vi "例7-6（1）.vi"() -> ()   [LabVIEW 2019]
uses:
  <vilib>/Analysis/NI_AALBase.lvlib
panel:
  in  "停止":bool
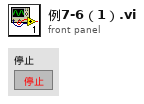
[diagram p1: front panel]
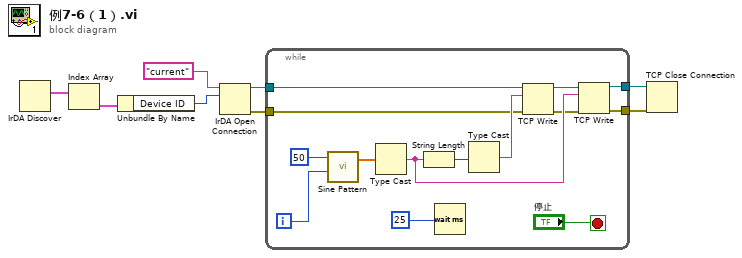
[diagram p0: block diagram]
diagram:
  n1 = IrDA Discover() -> (2:w8:cluster{"Device ID":u32, "Device Name":string}[])  [unwired: 1 in, 2 out]
  n2 = Index Array(array=w8) -> (element=w7:cluster{"Device ID":u32, "Device Name":string})  [unwired: 1 in]
  n3 = Unbundle By Name(w7) -> ("Device ID"=w6:u32)
  n4 = IrDA Open Connection(10:w6, 11:"current" ("服务名称")) -> (0:w2:errorcluster, 3:w4:refnum<k19>)  [unwired: 2 in]
  n5 = while {
    tunnel: w4 -> [w15]
    tunnel: [w13] -> w3
    tunnel: w2 -> [w12]
    tunnel: [w10] -> w1
    i -> [w20]
    stop <- "停止" stop-if-true
    n6 = call <vilib>:"Sine Pattern.vi"("phase(degrees)"=w20, "samples"=50) -> ("Sinusoidal Pattern"=w19:dbl[])  [unwired: 2 in, 1 out]
    n7 = Type Cast(x=w19) -> (*(type *) &x=w16:string)  [unwired: 1 in]
    n8 = String Length(string=w16) -> (length=w18:i32)
    n9 = Wait (ms)(milliseconds to wait=25) -> ()  [unwired: 1 out]
    n10 = Type Cast(x=w18) -> (*(type *) &x=w17:string)  [unwired: 1 in]
    n11 = TCP Write(connection ID=w15, data in=w17, error in (no error)=w12) -> (connection ID out=w14:refnum<k19>, error out=w11:errorcluster)  [unwired: 1 in, 1 out]
    n12 = TCP Write(connection ID=w14, data in=w16, error in (no error)=w11) -> (connection ID out=w13:refnum<k19>, error out=w10:errorcluster)  [unwired: 1 in, 1 out]
  }
  n13 = TCP Close Connection(connection ID=w3, error in (no error)=w1) -> ()  [unwired: 1 in, 2 out]
